vi "Create UDP Error.vi"(9 "source vi name":string, 11 "Error":T1) -> (1 "offset":i32, 3 "error out":errorcluster)   [LabVIEW 2017, in "UDP Transceiver.lvlib" / "UDP Transceiver.lvclass"]
uses:
  UDP Transceiver.lvclass
  Errors.ctl
  <vilib>/NI/Memory Manager/VIs/New Error Cluster Constant (512B).vi
  Library Name.vi
  <vilib>/NI/Memory Manager/Static Error Handling.lvlib
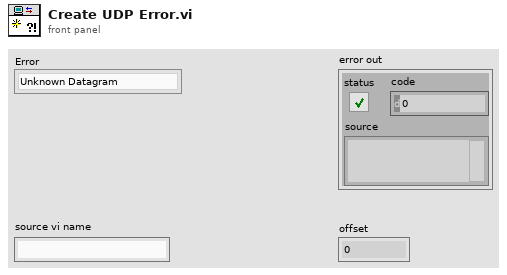
[diagram p1: front panel]
types:
  T1 = typedef "UDP Transceiver.lvlib/UDP Transceiver.lvclass/Errors.ctl" = enum16{"Unknown Datagram", "Size Mismatch"}
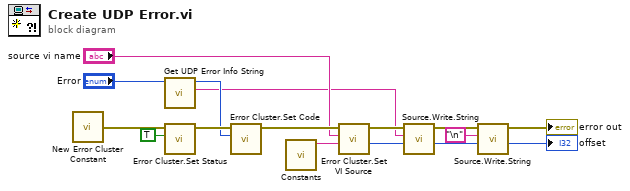
[diagram p0: block diagram]
diagram:
  n1 = call-poly <vilib>:"New Error Cluster Constant.vi"() -> ("error out"=w15:errorcluster)  [unwired: 1 in]
  n2 = call "Get UDP Error Info String.vi"("Error"="Error") -> ("description"=w6:string, "code"=w9:i32)  [unwired: 9 in]
  n3 = call <vilib>:"Error Cluster.Set Status.vi"("status (T)"=TRUE, "error in"=w15) -> ("error out"=w13:errorcluster)  [unwired: 9 in]
  n4 = call <vilib>:"Error Cluster.Set Code.vi"("code"=w9, "error in"=w13) -> ("error out"=w12:errorcluster)  [unwired: 9 in]
  n5 = call-poly "Constants.vi"() -> ("library name"=w10:string)  [unwired: 11 in]
  n6 = call <vilib>:"Error Cluster.Set VI Source.vi"("library name (\"\")"=w10, "vi name"="source vi name", "error in"=w12) -> ("new offset"=w7:i32, "error out"=w8:errorcluster)  [unwired: 7 in]
  n7 = call <vilib>:"Source.Write.String.vi"("offset"=w7, "string"=w6, "error in"=w8) -> ("new offset"=w4:i32, "error out"=w5:errorcluster)  [unwired: 7 in]
  n8 = call <vilib>:"Source.Write.String.vi"("offset"=w4, "string"="\n", "error in"=w5) -> ("new offset"=→"offset":i32, "error out"=→"error out":errorcluster)  [unwired: 7 in]
